vi "Tosca-Draw Grating.vi"(0 "Grating":T1, 7 "Array":cdb[][](array[numeric]), 9 "photodiode mask":u8[][](array[numeric])) -> (4 "RGB":u32[][](array[numeric]))   [LabVIEW 2020]
uses:
  Tosca-Grating.ctl
  Tosca-Grating Type.ctl
  epl-vi-lib/Utility VIs/Array Manipulation VIs/Array-Dimensions (2D).vi
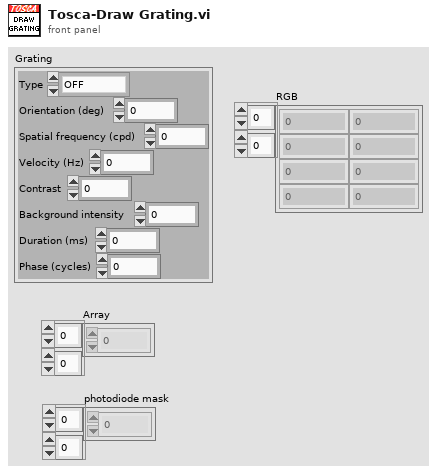
[diagram p1: front panel]
types:
  T1 = typedef "Tosca-Grating.ctl" = cluster{"Type":T2, "Orientation (deg)":dbl, "Spatial frequency (cpd)":dbl, "Velocity (Hz)":dbl, "Contrast":dbl, "Background intensity":dbl, "Duration (ms)":dbl, "Phase (cycles)":dbl}
  T2 = typedef "Tosca-Grating Type.ctl" = enum16{"OFF", "Square", "Sine"}
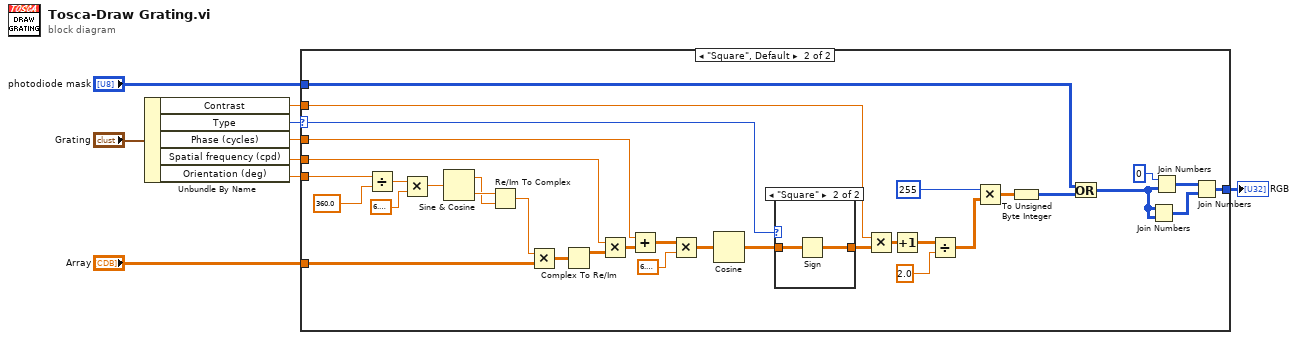
[diagram p0: block diagram]
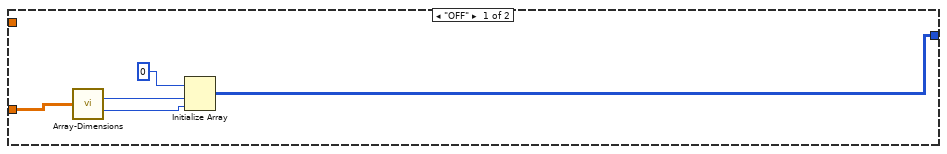
[diagram p2: hidden frame]
diagram:
  n1 = Unbundle By Name("Grating") -> ("Contrast"=w7:dbl, "Type"=w5:T2, "Phase (cycles)"=w1:dbl, "Spatial frequency (cpd)"=w8:dbl, "Orientation (deg)"=w3:dbl)
  n2 = case shown="\"Square\", Default" w5 {
    selector: w5 -> [_ w37]
    tunnel: w8 -> [_ w47]
    tunnel: w7 -> [_ w45]
    tunnel: [w10 w39] -> w6
    tunnel: "Array" -> [w14 w36]
    tunnel: w3 -> [_ w28]
    tunnel: "photodiode mask" -> [_ w18]
    tunnel: w1 -> [_ w15]
    frame "OFF" {
      n3 = call-poly "Array-Dimensions.vi"("2D Array"=w14) -> ("# rows"=w13:i32, "# columns"=w12:i32)  [unwired: 13 in]
      n4 = Initialize Array(u32 0, w13, w12) -> (w10:u32[][])
    }
    frame "Square", Default {
      n5 = Divide(x=w28, y=360.0) -> (x/y=w26:dbl)
      n6 = Multiply(x=w26, y=6.283185307179586) -> (x*y=w24:dbl)
      n7 = Sine & Cosine(0:w24) -> (1:w22:dbl, 2:w23:dbl)
      n8 = Re/Im To Complex(1:w22, 2:w23) -> (0:w20:cdb)
      n9 = Multiply(x=w20, y=w36) -> (x*y=w21:cdb[][])
      n10 = Complex To Re/Im(x + iy=w21) -> (x=w29:dbl[][])  [unwired: 1 out]
      n11 = Multiply(x=w47, y=w29) -> (x*y=w35:dbl[][])
      n12 = Add(x=w15, y=w35) -> (x+y=w16:dbl[][])
      n13 = Multiply(x=w16, y=6.283185307179586) -> (x*y=w34:dbl[][])
      n14 = Cosine(x=w34) -> (cos(x)=w33:dbl[][])
      n15 = case shown="\"Square\"" w37 {
        tunnel: w33 -> [w49 w51]
        tunnel: [w49 w50] -> w38
        frame "Sine", Default {
        }
        frame "Square" {
          n16 = Sign(1:w51) -> (0:w50:dbl[][])
        }
      }
      n17 = Multiply(x=w45, y=w38) -> (x*y=w44:dbl[][])
      n18 = Increment(x=w44) -> (x+1=w43:dbl[][])
      n19 = Divide(x=w43, y=2.0) -> (x/y=w40:dbl[][])
      n20 = Multiply(x=255, y=w40) -> (x*y=w48:dbl[][])
      n21 = To Unsigned Byte Integer(number=w48) -> (unsigned 8bit integer=w19:u8[][])
      n22 = Or(x=w18, y=w19) -> (x .or. y?=w17:u8[][])
      n23 = Join Numbers(hi=w17, lo=w17) -> ((hi.lo)=w32:u16[][])
      n24 = Join Numbers(hi=u8 0, lo=w17) -> ((hi.lo)=w31:u16[][])
      n25 = Join Numbers(hi=w31, lo=w32) -> ((hi.lo)=w39:u32[][])
    }
  }
  "RGB" <- w6
